vi "Save Waveform Memory.vi"(8 "error in (no error)":errorcluster, 9 "Waveform Memory (9: Memory 1)":u16(ring) items=["Memory 1", "Memory 2", "Memory 3", "Memory 4"], 10 "Channel (1: Channel 1)":u16(ring) items=["Channel 1", "Channel 2", "Channel 3", "Channel 4", "Function 1", "Function 2", "Function 3", "Function 4", "Memory 1", "Memory 2", "Memory 3", "Memory 4"], 11 "VISA resource name":refnum<visa-resource-name>) -> (0 "error out":errorcluster, 3 "VISA resource name out":refnum<visa-resource-name>)   [LabVIEW 2009, in "Agilent 8000 Series.lvlib"]
doc: "Stores the specified channel, waveform memory, or function to the waveform memory. The channel or function must be enabled or an error status is returned. User can save waveform to waveform memories whether the waveform memory is displayed or not."
uses:
  Agilent 8000 Series.lvlib
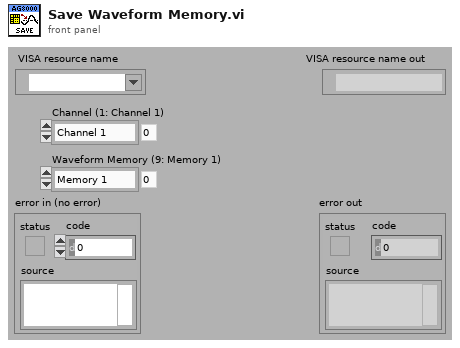
[diagram p1: front panel]
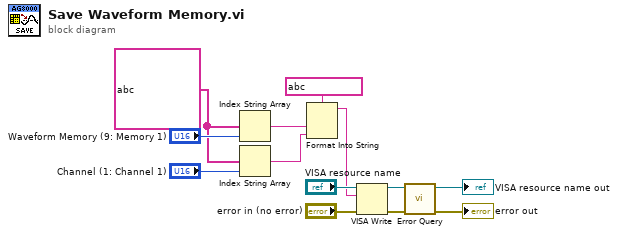
[diagram p0: block diagram]
diagram:
  w4 = string[] ?
  n1 = Index String Array(1:"Waveform Memory (9: Memory 1)", 2:w4) -> (0:w2:string)  [unwired: 1 in]
  n2 = Index String Array(1:"Channel (1: Channel 1)", 2:w4) -> (0:w3:string)  [unwired: 1 in]
  n3 = Format Into String(format string=string ?, w2, w3) -> (resulting string=w1:string)  [unwired: 2 in, 1 out]
  n4 = VISA Write(VISA resource name="VISA resource name", write buffer=w1, error in (no error)="error in (no error)") -> (VISA resource name out=w9:refnum<visa-resource-name>, error out=w8:errorcluster)  [unwired: 1 out]
  n5 = call "Error Query.vi"("error in (no error)"=w8, "VISA resource name"=w9) -> ("error out"=→"error out":errorcluster, "VISA resource name out"=→"VISA resource name out":refnum<visa-resource-name>)  [unwired: 6 in, 2 out]
